vi "setClaseVarilla.vi"(8 "error in":errorcluster, 10 "dataToSet":T1, 11 "claseVarilla in":refnum<class "claseVarilla.lvclass">) -> (0 "error out":errorcluster, 3 "claseVarilla out":refnum<class "claseVarilla.lvclass">)   [LabVIEW 2014, in "claseVarilla.lvclass"]
uses:
  claseVarilla.lvclass
  claseVarilla.lvclass/claseVarilla.ctl
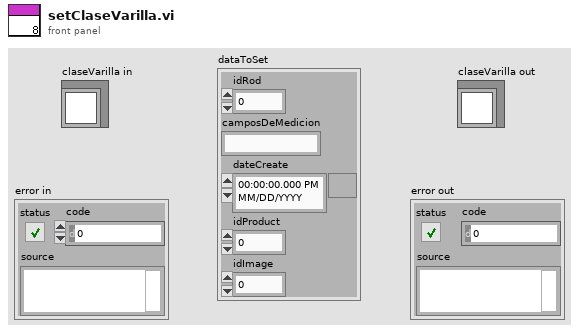
[diagram p1: front panel]
types:
  T1 = cluster{"idRod":dbl, "camposDeMedicion":string, "dateCreate":timestamp, "idProduct":dbl, "idImage":dbl}
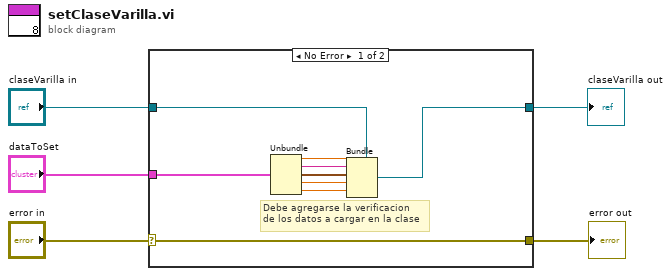
[diagram p0: block diagram]
diagram:
  n1 = case shown="No Error" "error in" {
    selector: "error in" -> [w14 w16]
    tunnel: [w14 w16] -> w4
    tunnel: [w12 w15] -> w3
    tunnel: "claseVarilla in" -> [w13 w15]
    tunnel: "dataToSet" -> [w9 _]
    frame No Error {
      # "Debe agregarse la verificacion \nde los datos a cargar en la clase"
      n2 = Unbundle(w9) -> ("idRod"=w11:dbl, "camposDeMedicion"=w10:string, "dateCreate"=w8:timestamp, "idProduct"=w7:dbl, "idImage"=w6:dbl)
      n3 = Bundle(cluster=w13, w11, w10, w8, w7, w6) -> (w12:refnum<class "claseVarilla.lvclass">)
    }
    frame Error {
    }
  }
  "claseVarilla out" <- w3
  "error out" <- w4
